vi "Evaluate Macro_Parameters.vi"(8 "Error In":errorcluster, 11 "Tree Refnum IN":refnum<vi>) -> (0 "Error Out":errorcluster, 2 "Macro Error":bool, 3 "Tree Refnum OUT":refnum<vi>)   [LabVIEW 2012]
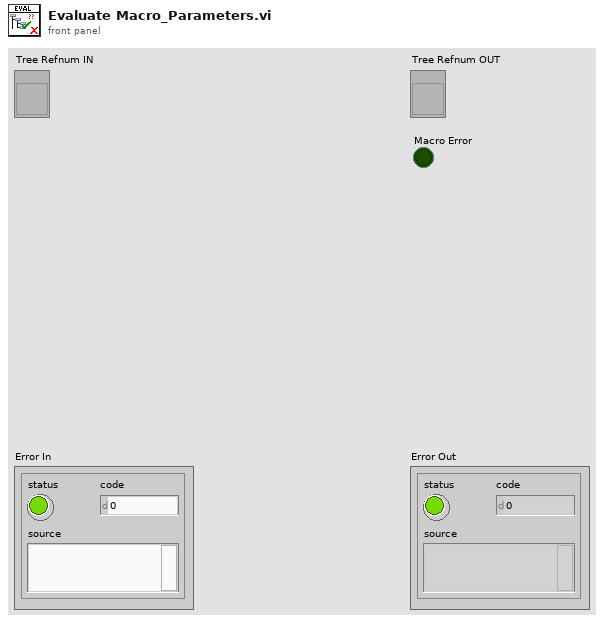
[diagram p1: front panel]
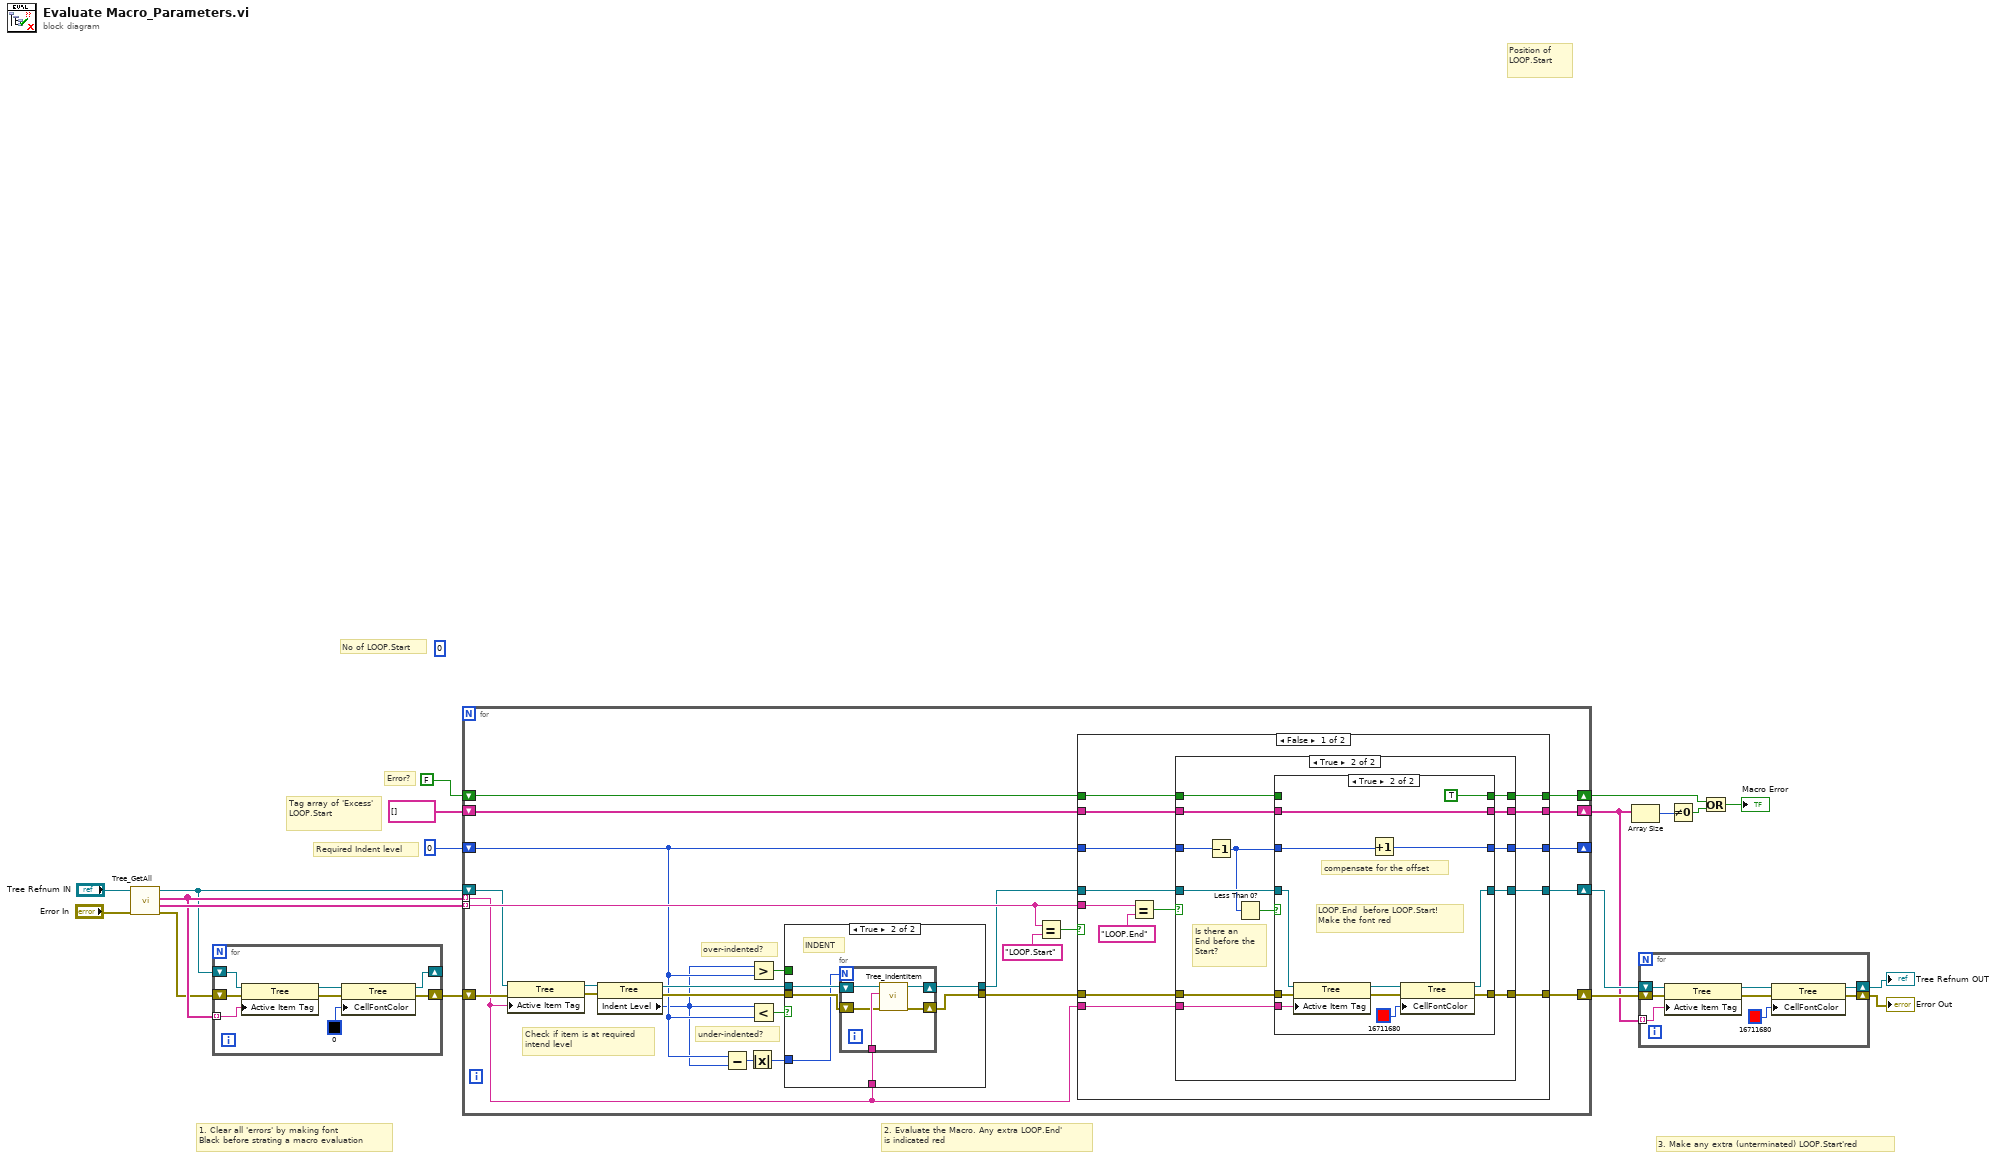
[diagram p0: block diagram]
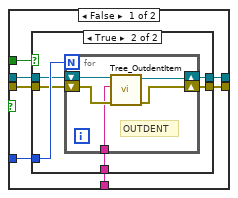
[diagram p2: hidden frame]
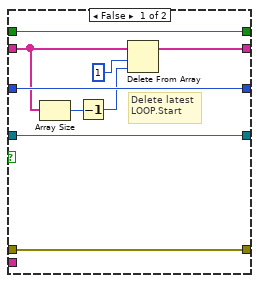
[diagram p5: hidden frame]
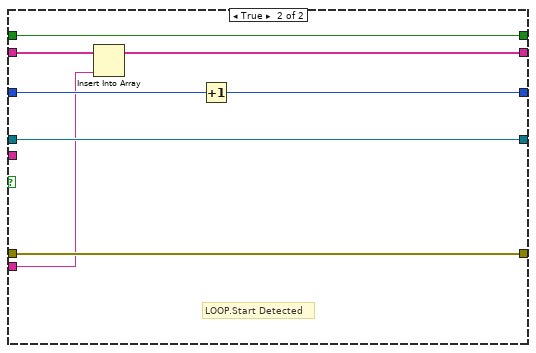
[diagram p6: hidden frame]
diagram:
  (unwired) 0 ("index")
  # "Error?"
  # "2. Evaluate the Macro. Any extra LOOP.End'\nis indicated red"
  # "3. Make any extra (unterminated) LOOP.Start'red"
  # "1. Clear all 'errors' by making font\nBlack before strating a macro evaluation"
  # "Tag array of 'Excess' LOOP.Start"
  # "Required Indent level"
  # "No of LOOP.Start"
  # "Position of LOOP.Start"
  n1 = call "Tree_GetAll.vi"("Error In"="Error In", "Tree Refnum IN"="Tree Refnum IN") -> ("Error Out"=w13:errorcluster, "Text"=w15:string[], "Tags"=w14:string[], "Tree Refnum OUT"=w12:refnum<vi>)  [unwired: 6 in]
  n2 = for {
    tunnel: w14 -> [w25] mode=indexing
    shift-right: [w22] -> w11
    shift-left: w13 -> [w27]
    shift-right: [w21] -> _
    shift-left: w12 -> [w26]
    n3 = property class="Tree"(reference=w26, error in=w27, "Active Item Tag"=w25) -> (reference out=w23:refnum<vi>, error out=w24:errorcluster)
    n4 = property class="Tree"(reference=w23, error in=w24, "CellFontColor"=u32 0) -> (reference out=w21:refnum<vi>, error out=w22:errorcluster)
  }
  n5 = for {
    tunnel: w15 -> [w51] mode=indexing
    shift-right: [w38] -> w10
    shift-left: w12 -> [w41]
    shift-right: [w42] -> _
    shift-left: 0 ("index") -> [w33]
    tunnel: w14 -> [w28] mode=indexing
    shift-right: [w37] -> w9
    shift-left: w11 -> [w34]
    shift-right: [w35] -> w6
    shift-left: string[] [] -> [w36]
    shift-right: [w30] -> w3
    shift-left: FALSE -> [w29]
    # "under-indented?"
    # "over-indented?"
    # "Check if item is at required\nintend level"
    n6 = property class="Tree"(reference=w41, error in=w34, "Active Item Tag"=w28) -> (reference out=w47:refnum<vi>, error out=w48:errorcluster)
    n7 = property class="Tree"(reference=w47, error in=w48) -> (reference out=w49:refnum<vi>, error out=w50:errorcluster, "Indent Level"=w32:i32)
    n8 = Subtract(x=w33, y=w32) -> (x-y=w44:i32)
    n9 = Absolute Value(x=w44) -> (abs(x)=w43:i32)
    n10 = Greater?(x=w32, y=w33) -> (0:w31:bool)
    n11 = Less?(x=w32, y=w33) -> (x < y?=w45:bool)
    n12 = case shown="True" w45 {
      tunnel: [w54 w78] -> w40
      tunnel: w28 -> [w55 w77]
      tunnel: [w53 w76] -> w39
      tunnel: w50 -> [w56 w75]
      tunnel: w49 -> [w57 w74]
      tunnel: w43 -> [w58 w73]
      tunnel: w31 -> [w59 _]
      frame False {
        n13 = case shown="True" w59 {
          tunnel: w58 -> [_ w67]
          tunnel: w57 -> [w61 w66]
          tunnel: w56 -> [w60 w65]
          tunnel: w55 -> [_ w64]
          tunnel: [w61 w63] -> w54
          tunnel: [w60 w62] -> w53
          frame False {
          }
          frame True {
            n14 = for {
              N: w67 -> [_]
              shift-right: [w69] -> w63
              shift-left: w66 -> [w70]
              shift-right: [w68] -> w62
              shift-left: w65 -> [w72]
              tunnel: w64 -> [w71]
              # "OUTDENT"
              n15 = call "Tree_OutdentItem.vi"("Error In"=w72, "TagToOutdent"=w71, "Tree Refnum"=w70) -> ("Error Out"=w68:errorcluster, "Tree Refnum OUT"=w69:refnum<vi>)  [unwired: 7 in]
            }
          }
        }
      }
      frame True {
        # "INDENT"
        n16 = for {
          N: w73 -> [_]
          tunnel: w77 -> [w82]
          shift-right: [w81] -> w76
          shift-left: w75 -> [w80]
          shift-right: [w83] -> w78
          shift-left: w74 -> [w79]
          n17 = call "Tree_IndentItem.vi"("Error In"=w80, "TagToIndent"=w82, "Tree Refnum"=w79) -> ("Error Out"=w81:errorcluster, "Tree Refnum OUT"=w83:refnum<vi>)  [unwired: 7 in]
        }
      }
    }
    n18 = Equal?(x=w51, y="LOOP.Start") -> (x = y?=w46:bool)
    n19 = case shown="False" w46 {
      tunnel: w40 -> [w92 w142]
      tunnel: w33 -> [w95 w144]
      tunnel: w51 -> [w96 _]
      tunnel: [w94 w143] -> w42
      tunnel: w28 -> [w93 w138]
      tunnel: [w91 w142] -> w38
      tunnel: w39 -> [w90 w141]
      tunnel: [w89 w141] -> w37
      tunnel: w36 -> [w87 w140]
      tunnel: [w86 w139] -> w35
      tunnel: [w85 w137] -> w30
      tunnel: w29 -> [w84 w137]
      frame False {
        n20 = Equal?(x=w96, y="LOOP.End") -> (x = y?=w88:bool)
        n21 = case shown="True" w88 {
          tunnel: w95 -> [w102 w108]
          tunnel: [w102 w115] -> w94
          tunnel: w93 -> [_ w114]
          tunnel: w92 -> [w101 w113]
          tunnel: [w101 w112] -> w91
          tunnel: w90 -> [w100 w111]
          tunnel: [w100 w110] -> w89
          tunnel: w87 -> [w99 w106]
          tunnel: [w99 w105] -> w86
          tunnel: [w98 w104] -> w85
          tunnel: w84 -> [w98 w103]
          frame False {
            # "Some other command\n- Do nothing"
          }
          frame True {
            # "Is there an \nEnd before the\nStart?"
            n22 = Decrement(x=w108) -> (x-1=w107:i32)
            n23 = Less Than 0?(x=w107) -> (x < 0?=w109:bool)
            n24 = case shown="True" w109 {
              tunnel: w107 -> [w122 w127]
              tunnel: [w122 w126] -> w115
              tunnel: w114 -> [_ w136]
              tunnel: w113 -> [w123 w132]
              tunnel: [w123 w131] -> w112
              tunnel: w111 -> [w124 w130]
              tunnel: [w124 w129] -> w110
              tunnel: w106 -> [w120 w128]
              tunnel: [w121 w128] -> w105
              tunnel: [w116 TRUE] -> w104
              tunnel: w103 -> [w116 _]
              frame False {
                # "Delete latest LOOP.Start"
                n25 = Array Size(array=w120) -> (size(s)=w119:i32)
                n26 = Decrement(x=w119) -> (x-1=w117:i32)
                n27 = Delete From Array(array=w120, length=1, index=w117) -> (array with subset deleted=w121:string[])  [unwired: 1 out]
              }
              frame True {
                # "compensate for the offset"
                # "LOOP.End  before LOOP.Start!\nMake the font red"
                n28 = property class="Tree"(reference=w132, error in=w130, "Active Item Tag"=w136) -> (reference out=w135:refnum<vi>, error out=w134:errorcluster)
                n29 = Increment(x=w127) -> (x+1=w126:i32)
                n30 = property class="Tree"(reference=w135, error in=w134, "CellFontColor"=u32 16711680) -> (reference out=w131:refnum<vi>, error out=w129:errorcluster)
              }
            }
          }
        }
      }
      frame True {
        # "LOOP.Start Detected"
        n31 = Insert Into Array(array=w140, new element=w138) -> (w139:string[])  [unwired: 1 in]
        n32 = Increment(x=w144) -> (x+1=w143:i32)
      }
    }
  }
  n33 = Array Size(array=w6) -> (size(s)=w5:i32)
  n34 = for {
    tunnel: w6 -> [w146] mode=indexing
    shift-right: [w147] -> w7
    shift-left: w9 -> [w148]
    shift-right: [w145] -> w8
    shift-left: w10 -> [w149]
    n35 = property class="Tree"(reference=w149, error in=w148, "Active Item Tag"=w146) -> (reference out=w150:refnum<vi>, error out=w151:errorcluster)
    n36 = property class="Tree"(reference=w150, error in=w151, "CellFontColor"=u32 16711680) -> (reference out=w145:refnum<vi>, error out=w147:errorcluster)
  }
  "Error Out" <- w7
  "Tree Refnum OUT" <- w8
  n37 = Not Equal To 0?(x=w5) -> (x != 0?=w4:bool)
  n38 = Or(x=w3, y=w4) -> (x .or. y?=→"Macro Error":bool)
